vi "3P_Wait.vi"(0 "Parallel Task in":refnum<k21>, 5 "P task error in":errorcluster, 9 "NHR VISA in":refnum<visa-resource-name>, 11 "NHR error in":errorcluster caption="NHR error in (no error)", 12 "Wait Filepath":path=path "C:/Users/ga11/Desktop/VI/results/3PtestChrgRest.lvm" caption="Filename", 13 "Wait time":dbl) -> (2 "WaitElapsed Time (s)":i32 caption="Elapsed Time (s)", 4 "parallel task out":refnum<k21>, 6 "parallel task error out":errorcluster, 10 "NHR Visa Out":refnum<visa-resource-name>, 15 "NHR error out":errorcluster)   [LabVIEW 2020]
uses:
  <vilib>/DAQmx/read.llb/DAQmx Read (Analog 1D DBL NChan 1Samp).vi
  <vilib>/DAQmx/miscellaneous.llb/DAQmx Fill In Error Info.vi
  <instrlib>/NH Research Regenerative Test Series/Public/Data/Read (Ave Current).vi
  <instrlib>/NH Research Regenerative Test Series/Public/Data/Low Level/Fetch (Ave Voltage).vi
  <instrlib>/NH Research Regenerative Test Series/Public/Data/Low Level/Fetch (Ave True Power).vi
  <instrlib>/NH Research Regenerative Test Series/NH Research Regenerative Test Series.lvlib
panel:
  out "Ave Current (A) 2":dbl
  out "Ave Voltage (V) 2":dbl
  out "Ave True Power (W) 2":dbl
  out "Status Byte Register 2":T1
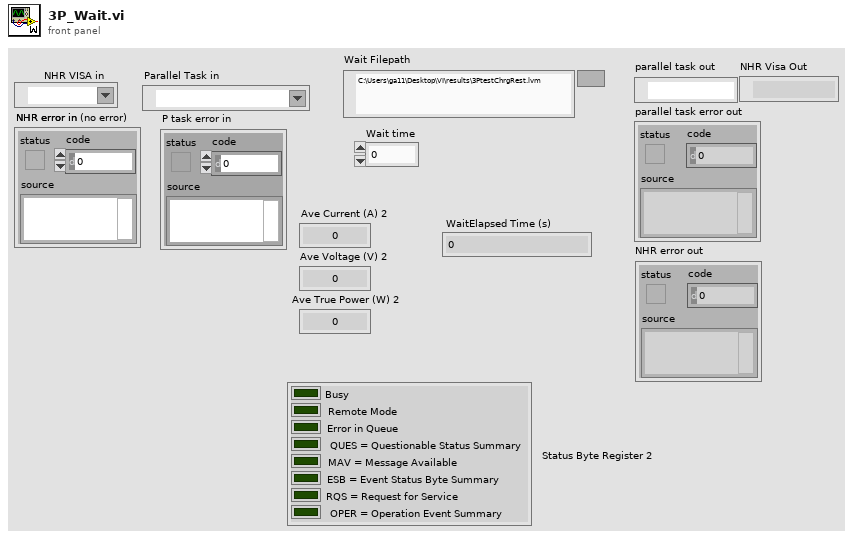
[diagram p1: front panel]
types:
  T1 = cluster{"Busy":bool, "Remote Mode":bool, "Error in Queue":bool, "QUES = Questionable Status Summary":bool, "MAV = Message Available":bool, "ESB = Event Status Byte Summary":bool, "RQS = Request for Service":bool, "OPER = Operation Event Summary":bool}
  T2 = cluster{"data[0]":dbl, "data[1]":dbl, "data[2]":dbl, "data[3]":dbl, "data[4]":dbl, "data[5]":dbl, "data[6]":dbl, "data[7]":dbl, "data[8]":dbl, "data[9]":dbl}
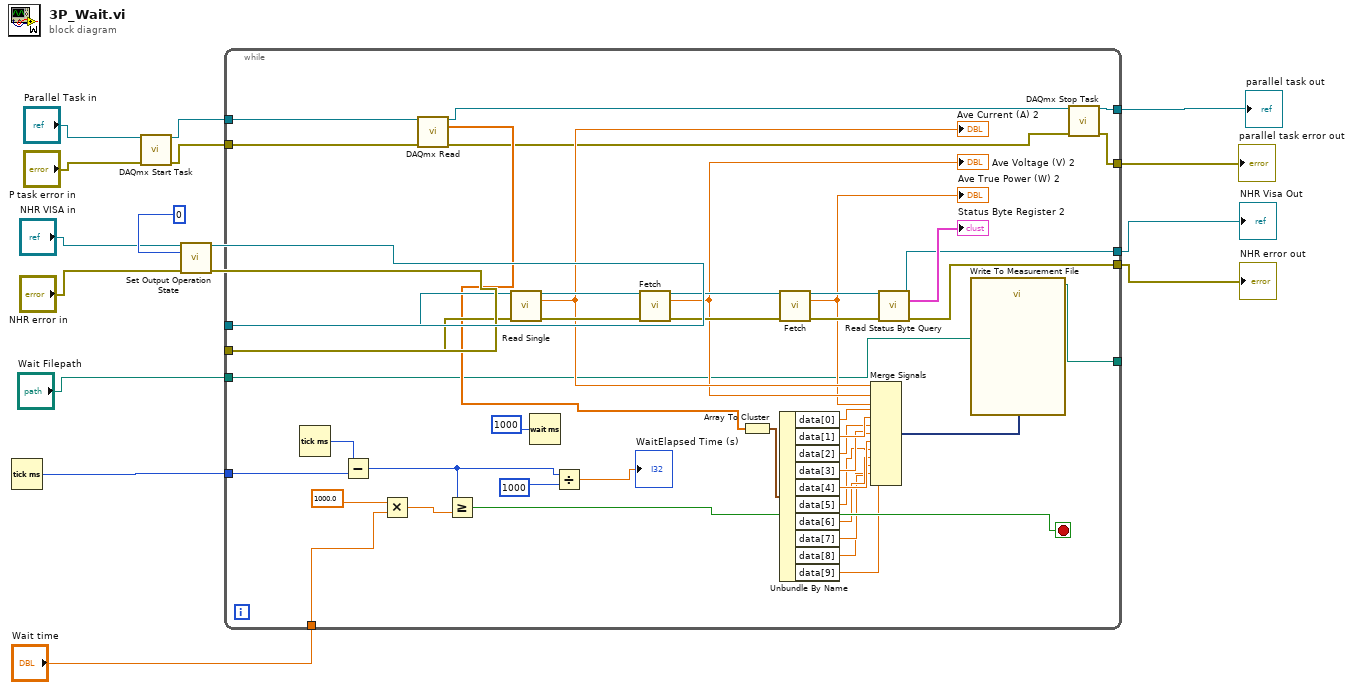
[diagram p0: block diagram]
diagram:
  n1 = Tick Count (ms)() -> (millisecond timer value=w10:u32)
  n2 = call <vilib>:"DAQmx Start Task.vi"("task/channels in"="Parallel Task in", "error in"="P task error in") -> ("task out"=w12:refnum<k21>, "error out"=w11:errorcluster)  [unwired: 12 in]
  n3 = call <vilib>:"Set Output Operation State.vi"("VISA resource name"="NHR VISA in", "Mode (0: Off)"=0, "error in (no error)"="NHR error in") -> ("VISA resource name out"=w15:refnum<visa-resource-name>, "error out"=w14:errorcluster)  [unwired: 11 in]
  n4 = while {
    tunnel: w15 -> [w54]
    tunnel: w14 -> [w53]
    tunnel: [w51] -> w9
    tunnel: [w50] -> w8
    tunnel: "Wait time" -> [w39]
    tunnel: [w36] -> _
    tunnel: w12 -> [w27]
    tunnel: w11 -> [w26]
    tunnel: w10 -> [w25]
    tunnel: "Wait Filepath" -> [w24]
    tunnel: [w21] -> w2
    tunnel: [w20] -> w1
    stop <- w40 stop-if-true
    n5 = Tick Count (ms)() -> (millisecond timer value=w41:u32)
    n6 = Subtract(x=w41, y=w25) -> (x-y=w19:u32)
    n7 = Multiply(x=1000.0, y=w39) -> (x*y=w37:dbl)
    n8 = call-poly <vilib>:"DAQmx Read.vi"("task/channels in"=w27, "error in"=w26) -> ("task out"=w23:refnum<k21>, "data"=w46:dbl[], "error out"=w22:errorcluster)  [unwired: 11 in]
    n9 = Greater Or Equal?(x=w19, y=w37) -> (x >= y?=w40:bool)
    n10 = call-poly <instrlib>:"Read Single.vi"("VISA resource name"=w54, "error in (no error)"=w53) -> ("VISA resource name out"=w59:refnum<visa-resource-name>, "Ave Current (A)"=w49:dbl, "error out"=w60:errorcluster)  [unwired: 11 in]
    "Ave Current (A) 2" <- w49
    n11 = Wait (ms)(milliseconds to wait=1000) -> ()  [unwired: 1 out]
    n12 = Divide(x=w19, y=1000) -> (x/y=→"WaitElapsed Time (s)":dbl)
    n13 = call-poly <instrlib>:"Fetch.vi"("VISA resource name"=w59, "error in (no error)"=w60) -> ("VISA resource name out"=w58:refnum<visa-resource-name>, "Ave Voltage (V)"=w48:dbl, "error out"=w57:errorcluster)  [unwired: 11 in]
    "Ave Voltage (V) 2" <- w48
    n14 = Array To Cluster(array=w46) -> (cluster=w45:T2)
    n15 = call-poly <instrlib>:"Fetch.vi"("VISA resource name"=w58, "error in (no error)"=w57) -> ("VISA resource name out"=w56:refnum<visa-resource-name>, "Ave True Power (W)"=w47:dbl, "error out"=w55:errorcluster)  [unwired: 11 in]
    "Ave True Power (W) 2" <- w47
    n16 = Unbundle By Name(w45) -> ("data[0]"=w44:dbl, "data[1]"=w43:dbl, "data[2]"=w35:dbl, "data[3]"=w34:dbl, "data[4]"=w33:dbl, "data[5]"=w32:dbl, "data[6]"=w31:dbl, "data[7]"=w30:dbl, "data[8]"=w29:dbl, "data[9]"=w28:dbl)
    n17 = Merge Signals "Merge Signals"(w49, w48, w47, w44, w43, w35, w34, w33, w32, w31, w30, w29, w28) -> (w61:dynamicdata)
    n18 = call <instrlib>:"Read Status Byte Query.vi"("VISA resource name"=w56, "error in (no error)"=w55) -> ("VISA resource name out"=w51:refnum<visa-resource-name>, "Status Byte Register"=→"Status Byte Register 2":T1, "error out"=w50:errorcluster)  [unwired: 11 in]
    n19 = call "Write To Measurement File"("Signals"=w61, "Filename"=w24) -> ("Filename Out"=w36:path)  [unwired: 15 in, 2 out]
    n20 = call <vilib>:"DAQmx Stop Task.vi"("task/channels in"=w23, "error in"=w22) -> ("task out"=w21:refnum<k21>, "error out"=w20:errorcluster)  [unwired: 12 in]
  }
  "parallel task out" <- w2
  "parallel task error out" <- w1
  "NHR Visa Out" <- w9
  "NHR error out" <- w8
